vi "Create buffer for strings.vi"(4 "# of spaces":i32) -> (1 "String Buffer":string)   [LabVIEW 2015]
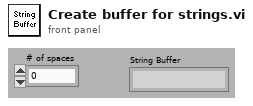
[diagram p1: front panel]
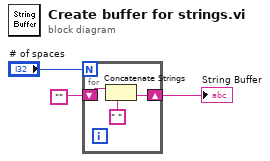
[diagram p0: block diagram]
diagram:
  n1 = for {
    N: "# of spaces" -> [_]
    shift-right: [w5] -> w2
    shift-left: "" -> [w4]
    n2 = Concatenate Strings(w4, " ") -> (w5:string)
  }
  "String Buffer" <- w2
